vi "Wave2D_Init Sol.vi"(10 "Boundary Condition":cluster{"type":T2, "Value":dbl[][]}[](array[cluster]) {"type" items=["Dirichlet", "Neumann"]}, 11 "Domain":T1={"t"={"initial t"=0.0, "final t"=1.0, "# of t-points"=11}, "x"={"start x"=0.0, "end x"=1.0, "# of x-points"=11}, "y"={"start y"=0.0, "end y"=1.0, "# of y-points"=11}}) -> (3 "U(t, x, y)":dbl[][][](array[numeric]))   [LabVIEW 2017, in "NI_PDE.lvlib"]
uses:
  <vilib>/gmath/NI_PDE.lvlib
  <vilib>/gmath/pde.llb/Common/PDE_BC Type.ctl
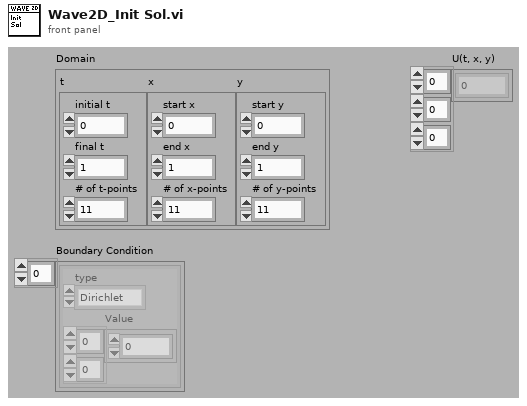
[diagram p1: front panel]
types:
  T1 = cluster{"t":cluster{"initial t":dbl, "final t":dbl, "# of t-points":i32}, "x":cluster{"start x":dbl, "end x":dbl, "# of x-points":i32}, "y":cluster{"start y":dbl, "end y":dbl, "# of y-points":i32}}
  T2 = typedef "NI_PDE.lvlib/PDE_BC Type.ctl" = i32
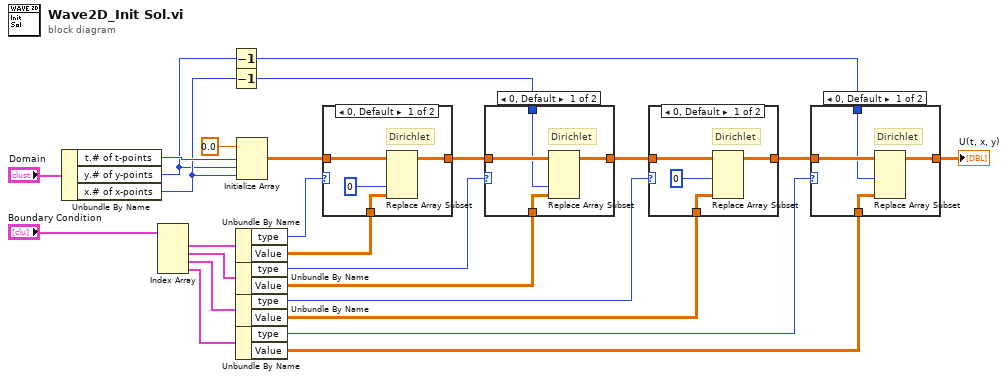
[diagram p0: block diagram]
diagram:
  n1 = Unbundle By Name("Domain") -> ("t.# of t-points"=w7:i32, "y.# of y-points"=w2:i32, "x.# of x-points"=w4:i32)
  n2 = Index Array(array="Boundary Condition") -> (element #1=w24:cluster{"type":T2, "Value":dbl[][]}, element #2=w23:cluster{"type":T2, "Value":dbl[][]}, element #3=w22:cluster{"type":T2, "Value":dbl[][]}, element #4=w21:cluster{"type":T2, "Value":dbl[][]})  [unwired: 4 in]
  n3 = Decrement(x=w2) -> (x-1=w1:i32)
  n4 = Decrement(x=w4) -> (x-1=w3:i32)
  n5 = Unbundle By Name(w24) -> ("type"=w20:T2, "Value"=w19:dbl[][])
  n6 = Unbundle By Name(w23) -> ("type"=w17:T2, "Value"=w16:dbl[][])
  n7 = Unbundle By Name(w22) -> ("type"=w15:T2, "Value"=w14:dbl[][])
  n8 = Unbundle By Name(w21) -> ("type"=w12:T2, "Value"=w10:dbl[][])
  n9 = Initialize Array(0.0 ("element"), w7, w2, w4) -> (w5:dbl[][][])
  n10 = case shown="0, Default" w20 {
    tunnel: w5 -> [w29 w30]
    tunnel: [w28 w30] -> w18
    tunnel: w19 -> [w27 _]
    frame 0, Default {
      # "Dirichlet"
      n11 = Replace Array Subset(array=w29, new element=w27, index (dim 2)=0 ("disabled index (row)")) -> (w28:dbl[][][])  [unwired: 2 in]
    }
    frame 1 {
    }
  }
  n12 = case shown="0, Default" w17 {
    tunnel: w18 -> [w34 w35]
    tunnel: [w33 w35] -> w13
    tunnel: w16 -> [w32 _]
    tunnel: w3 -> [w31 _]
    frame 0, Default {
      # "Dirichlet"
      n13 = Replace Array Subset(array=w34, new element=w32, index (dim 2)=w31) -> (w33:dbl[][][])  [unwired: 2 in]
    }
    frame 1 {
    }
  }
  n14 = case shown="0, Default" w15 {
    tunnel: w13 -> [w39 w40]
    tunnel: [w38 w40] -> w11
    tunnel: w14 -> [w37 _]
    frame 0, Default {
      # "Dirichlet"
      n15 = Replace Array Subset(array=w39, new element=w37, index (dim 1)=0 ("disabled index (row)")) -> (w38:dbl[][][])  [unwired: 2 in]
    }
    frame 1 {
    }
  }
  n16 = case shown="0, Default" w12 {
    tunnel: w11 -> [w44 w45]
    tunnel: [w43 w45] -> w9
    tunnel: w10 -> [w42 _]
    tunnel: w1 -> [w41 _]
    frame 0, Default {
      # "Dirichlet"
      n17 = Replace Array Subset(array=w44, new element=w42, index (dim 1)=w41) -> (w43:dbl[][][])  [unwired: 2 in]
    }
    frame 1 {
    }
  }
  "U(t, x, y)" <- w9
